vi "client_FGV 2.vi"(7 "data in":string, 8 "error constant":errorcluster, 9 "port":u16=6340, 10 "address":string="127.0.0.1", 11 "Enum":enum16{"open", "idle", "write", "read", "close"}(ring)) -> (0 "error constant 2":errorcluster, 3 "data out":string)   [LabVIEW 2015]
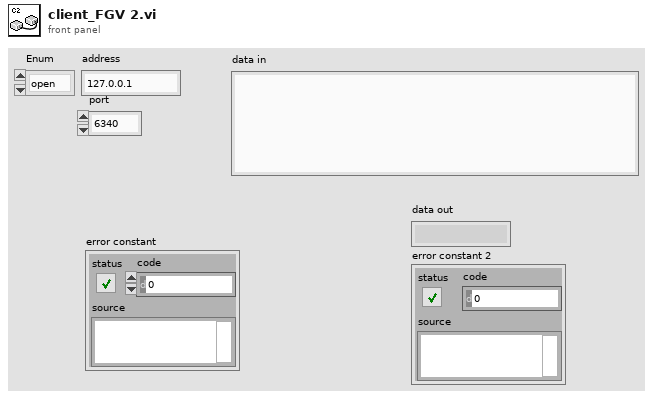
[diagram p1: front panel]
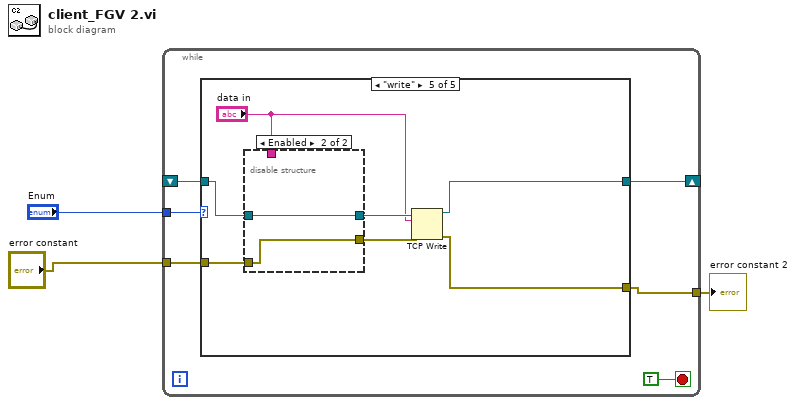
[diagram p0: block diagram]
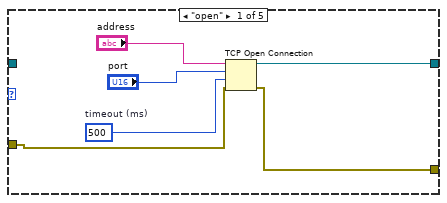
[diagram p2: hidden frame]
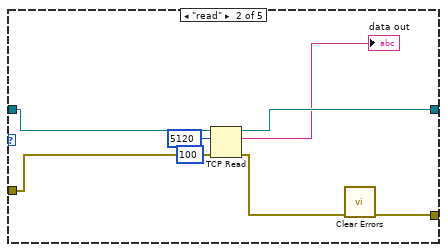
[diagram p3: hidden frame]
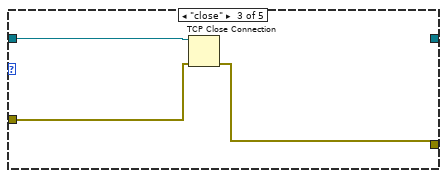
[diagram p4: hidden frame]
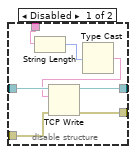
[diagram p6: hidden frame]
diagram:
  n1 = while {
    tunnel: "Enum" -> [w9]
    shift-right: [w8] -> _
    shift-left: _ -> [w7]
    tunnel: "error constant" -> [w6]
    tunnel: [w5] -> w1
    stop <- TRUE stop-if-true
    n2 = case shown="\"write\"" w9 {
      tunnel: [w13 w22 _ w28 w30] -> w8
      tunnel: w7 -> [_ w23 w26 w28 w32]
      tunnel: w6 -> [w11 w20 w25 w27 w35]
      tunnel: [w12 w18 w24 w27 w33] -> w5
      frame "open" {
        w15 = 500  # timeout (ms)
        n3 = TCP Open Connection(address="address", remote port or service name="port", timeout ms (60000)=w15, error in (no error)=w11) -> (connection ID=w13:refnum<k5>, error out=w12:errorcluster)  [unwired: 1 in]
      }
      frame "read" {
        n4 = TCP Read(connection ID=w23, bytes to read=5120, error in (no error)=w20, 9:100 ("timeout ms (25000)")) -> (connection ID out=w22:refnum<k5>, data out=→"data out":string, error out=w17:errorcluster)  [unwired: 1 out]
        n5 = call <vilib>:"Clear Errors.vi"("error in (no error)"=w17) -> ("error out"=w18:errorcluster)  [unwired: 5 in, 1 out]
      }
      frame "close" {
        n6 = TCP Close Connection(connection ID=w26, error in (no error)=w25) -> (error out=w24:errorcluster)  [unwired: 1 in, 1 out]
      }
      frame "idle", Default {
      }
      frame "write" {
        n7 = disable-structure shown="Enabled" {
          disable-tunnel: w35 -> [w42 w43]
          disable-tunnel: [w41 w43] -> w34
          disable-tunnel: w32 -> [w40 w44]
          disable-tunnel: [w39 w44] -> w31
          disable-tunnel: "data in" -> [w38 _]
          frame Disabled {
            n8 = String Length(string=w38) -> (length=w37:i32)
            n9 = Type Cast(x=w37) -> (*(type *) &x=w36:string)  [unwired: 1 in]
            n10 = TCP Write(connection ID=w40, data in=w36, error in (no error)=w42) -> (connection ID out=w39:refnum<k5>, error out=w41:errorcluster)  [unwired: 1 in, 1 out]
          }
          frame Enabled {
          }
        }
        n11 = TCP Write(connection ID=w31, data in="data in", error in (no error)=w34) -> (connection ID out=w30:refnum<k5>, error out=w33:errorcluster)  [unwired: 1 in, 1 out]
      }
    }
  }
  "error constant 2" <- w1
